vi "Get SheetData.vi"(8 "error in":errorcluster, 11 "Worksheet in":refnum<k24>) -> (0 "error out":errorcluster, 2 "SheetData":refnum<k24>, 3 "Worksheet out":refnum<k24>)   [LabVIEW 2021, in "Open Xml.lvlib"]
uses:
  Open Xml.lvlib
  D:/git/Open-Xml-LabVIEW/dll/DocumentFormat.OpenXml.dll
  dll/DocumentFormat.OpenXml.dll
  D:/git/Open-Xml-LabVIEW/dll/DocumentFormat.OpenXml.Framework.dll
  dll/DocumentFormat.OpenXml.Framework.dll
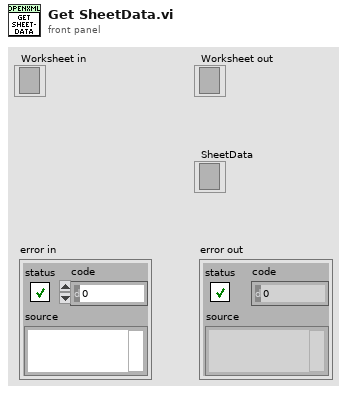
[diagram p1: front panel]
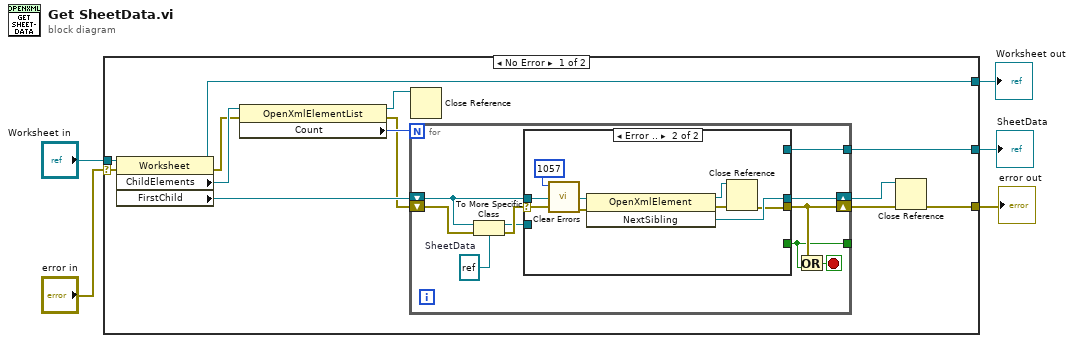
[diagram p0: block diagram]
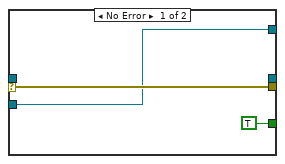
[diagram p2: hidden frame]
diagram:
  n1 = case shown="No Error" "error in" {
    selector: "error in" -> [w17 w41]
    tunnel: "Worksheet in" -> [w18 w40]
    tunnel: [w16 _] -> w3
    tunnel: [w7 w41] -> w2
    tunnel: [w10 w40] -> w1
    frame No Error {
      n2 = property class="Worksheet"(reference=w18, error in=w17) -> (reference out=w10:refnum<k24>, error out=w11:errorcluster, "ChildElements"=w13:refnum<k24>, "FirstChild"=w14:refnum<k24>)
      n3 = property class="OpenXmlElementList"(reference=w13, error in=w11) -> (reference out=w8:refnum<k24>, error out=w9:errorcluster, "Count"=w12:i32)
      n4 = for "Find SheetData" {
        N: w12 -> [_]
        shift-right: [w23] -> w6
        shift-left: w14 -> [w26]
        tunnel: [w24] -> w16
        shift-right: [w20] -> w15
        shift-left: w9 -> [w22]
        tunnel: [w19] -> _
        stop <- w21 stop-if-true
        w27 = refnum<k24> refnum  # SheetData
        n5 = To More Specific Class(target class=w27, reference=w26, error in=w22) -> (specific class reference=w25:refnum<k24>, error out=w28:errorcluster)
        n6 = case shown="Error .." w28 {
          selector: w28 -> [w31 w36]
          tunnel: [w31 w32] -> w20
          tunnel: [_ w39] -> w23
          tunnel: [TRUE _] -> w19
          tunnel: w26 -> [_ w38]
          tunnel: w25 -> [w29 _]
          tunnel: [w29 _] -> w24
          frame No Error {
          }
          frame Error {
            n7 = call <vilib>:"Clear Errors.vi"("error in (no error)"=w36, "specific error code to clear (0: all)"=1057) -> ("error out"=w35:errorcluster)  [unwired: 4 in, 1 out]
            n8 = invoke class="OpenXmlElement" method="NextSibling"(reference=w38, error in=w35) -> (reference out=w37:refnum<k24>, error out=w33:errorcluster, "NextSibling"=w39:refnum<k24>)  [unwired: 1 in]
            n9 = Close Reference(reference=w37, error in (no error)=w33) -> (error out=w32:errorcluster)
          }
        }
        n10 = Or(x=w20, y=w19) -> (x .or. y?=w21:bool)
      }
      n11 = Close Reference(reference=w8) -> ()  [unwired: 1 in, 1 out]
      n12 = Close Reference(reference=w6, error in (no error)=w15) -> (error out=w7:errorcluster)
    }
    frame Error {
    }
  }
  "error out" <- w2
  "SheetData" <- w3
  "Worksheet out" <- w1
